vi "Read Serial Porl.vi"(8 "error in (no error)":errorcluster, 11 "VISA Refnum in":refnum<visa-resource-name>) -> (0 "error out":errorcluster, 1 "read buffer":string, 2 "Array":dbl[](array[numeric]), 3 "VISA Refnum  out":refnum<visa-resource-name>)   [LabVIEW 2020]
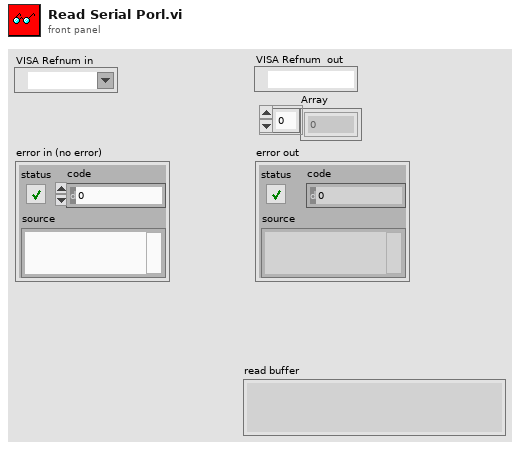
[diagram p1: front panel]
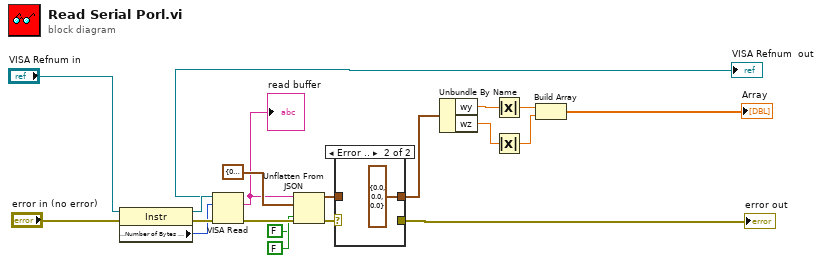
[diagram p0: block diagram]
diagram:
  n1 = property class="Instr"(reference="VISA Refnum in", error in="error in (no error)") -> (reference out=w14:refnum<visa-resource-name>, error out=w16:errorcluster, "Serial Settings:Number of Bytes at Serial Port"=w15:u32)
  n2 = VISA Read(VISA resource name=w14, byte count=w15, error in (no error)=w16) -> (VISA resource name out=→"VISA Refnum  out":refnum<visa-resource-name>, read buffer=w2:string, error out=w19:errorcluster)  [unwired: 1 out]
  "read buffer" <- w2
  n3 = Unflatten From JSON(JSON string=w2, type and defaults=cluster{"wx":dbl, "wy":dbl, "wz":dbl} {"wx"=0.0, "wy"=0.0, "wz"=0.0}, default null elements? (F)=FALSE, strict validation? (F)=FALSE, error in (no error)=w19) -> (value=w5:cluster{"wx":dbl, "wy":dbl, "wz":dbl}, error out=w3:errorcluster)  [unwired: 2 in]
  n4 = case shown="Error .." w3 {
    selector: w3 -> [w21 _]
    tunnel: [w22 cluster{"wx":dbl, "wy":dbl, "wz":dbl} {"wx"=0.0, "wy"=0.0, "wz"=0.0}] -> w4
    tunnel: w5 -> [w22 _]
    tunnel: [w21 _] -> w13
    frame No Error {
    }
    frame Error {
    }
  }
  "error out" <- w13
  n5 = Unbundle By Name(w4) -> ("wy"=w7:dbl, "wz"=w6:dbl)
  n6 = Absolute Value(x=w7) -> (abs(x)=w11:dbl)
  n7 = Absolute Value(x=w6) -> (abs(x)=w10:dbl)
  n8 = Build Array(w11, w10) -> (→"Array":dbl[])
